vi "HDF5_append-dataset-Test4vi.vi"() -> ()   [LabVIEW 2018]
uses:
  <vilib>/addons/h5labview2/file/H5F.lvlib
  <vilib>/addons/h5labview2/file/H5Fmode.ctl
  <vilib>/addons/h5labview2/dataset/H5D.lvlib
  HDF5/HDF5_ToneInfoClust.ctl
  <vilib>/addons/h5labview2/dataset/H5Dwrite.llb/H5Dwrite.xnode
  <vilib>/addons/h5labview2/space/H5S.lvlib
  <vilib>/addons/h5labview2/base/H5Equery.vi
  HDF5/lib_path_mod_20200519.vi
  <vilib>/addons/h5labview2/dataset/H5Dread.llb/H5Dread.xnode
  <vilib>/addons/h5labview2/base/hid_t_renamed.ctl
panel:
  out "data 2":T1[](array[typedef])
  in  "data":i32[][](array[numeric])=[[0, 1, 2, 3, 4], [5, 6, 7, 8, 9]]
  out "ms/append":dbl
  out "timer (ms)":u32
  out "progress":i32(slide)=9999 scale=0.0..10.0
  in  "repetitions":i32=10
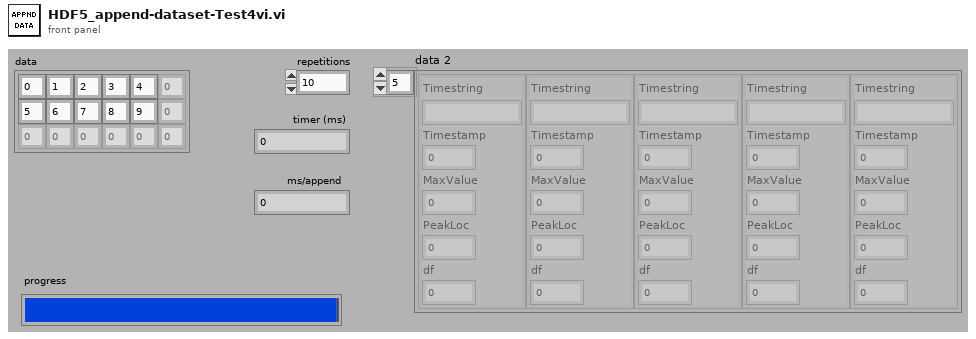
[diagram p1: front panel]
types:
  T1 = typedef "HDF5_ToneInfoClust.ctl" = cluster{"Timestring":string, "Timestamp":dbl, "MaxValue":dbl, "PeakLoc":dbl, "df":dbl}
  T2 = typedef "H5F.lvlib/H5Fmode.ctl" = enum16{"read-only", "read-write", "overwrite", "create new", "open or create"}
  T3 = typedef "HDF5_ToneInfoClust.ctl" = cluster{"Timestring":string, "Timestamp":timestamp, "MaxValue":dbl, "PeakLoc":dbl, "df":dbl}
  T4 = typedef "hid_t.ctl" = i32
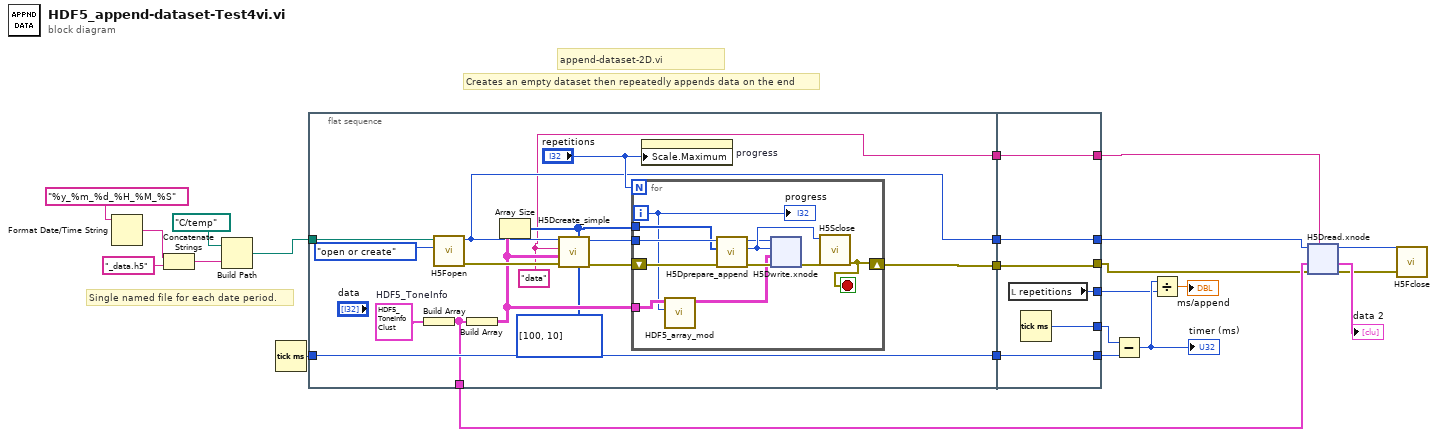
[diagram p0: block diagram]
diagram:
  # "Single named file for each date period."
  # "Creates an empty dataset then repeatedly appends data on the end"
  # "append-dataset-2D.vi"
  n1 = Format Date/Time String(time format string (%c)="%y_%m_%d_%H_%M_%S") -> (date/time string=w13:string)  [unwired: 2 in]
  n2 = Concatenate Strings(w13, "_data.h5" ("string")) -> (w15:string)
  n3 = Build Path(base path=path "C:/temp", name or relative path=w15) -> (appended path=w11:path)
  n4 = Tick Count (ms)() -> (millisecond timer value=w23:u32)
  n5 = flat-sequence {
    tunnel: w23 -> [w34]
    tunnel: [w34] -> w22
    tunnel: w11 -> [w32]
    tunnel: [w28] -> w9
    tunnel: [w27] -> w7
    tunnel: [w26] -> w6
    tunnel: [w25] -> w3
    tunnel: w22 -> [w73]
    tunnel: [w74] -> w21
    tunnel: [w73] -> w20
    tunnel: [w72] -> w18
    tunnel: [w71] -> w10
    tunnel: w9 -> [w71]
    tunnel: [w70] -> w8
    tunnel: w7 -> [w70]
    tunnel: [w69] -> w2
    tunnel: w3 -> [w69]
    frame #0 {
      w31 = T3 {"Timestring"="Timestamp string goes here", "Timestamp"=timestamp(0 s since 1904-01-01), "MaxValue"=0.0, "PeakLoc"=0.0, "df"=0.0}  # HDF5_ToneInfo
      w27 = "data" ("name")
      n6 = Build Array(w31) -> (w26:T3[])
      n7 = call <vilib>:"H5Fopen.vi"("mode (read-only)"=H5Fmode."open or create" ("mode"), "path"=w32) -> ("error out"=w35:errorcluster, "ref out"=w28:T4)  [unwired: 8 in]
      n8 = Build Array(w26) -> (w30:T3[][])
      n9 = Array Size(array=w30) -> (size(s)=w29:i32[])
      n10 = call <vilib>:"H5Dcreate_simple.vi"("max size"=u64[] [100, 10], "chunk size"=w29, "error in (no error)"=w35, "type in"=w30, "name"=w27, "ref in"=w28) -> ("error out"=w36:errorcluster, "dset out"=w37:T4)  [unwired: 4 in]
      n11 = for {
        N: "repetitions" -> [_]
        shift-right: [w45] -> w25
        shift-left: w36 -> [w46]
        tunnel: w29 -> [w47]
        tunnel: w37 -> [w48]
        tunnel: w30 -> [w41]
        i -> [w39]
        stop <- w45 stop-if-true
        n12 = call "HDF5_array_mod.vi"("delta"=w39, "Array in"=w41) -> ("Array out"=w40:T1[][])  [unwired: 9 in]
        n13 = call <vilib>:"H5Dprepare_append.vi"("error in (no error)"=w46, "append dims"=w47, "dset in"=w48) -> ("error out"=w49:errorcluster, "space out"=w43:T4, "dset out"=w42:T4)  [unwired: 5 in, 1 out]
        n14 = xnode "H5Dwrite.xnode"("error in (no error)"=w49, "data"=w40, "file space"=w43, "ref in"=w42) -> ("error out"=w44:errorcluster)  [unwired: 3 in, 2 out]
        n15 = call <vilib>:"H5Sclose.vi"("error in (no error)"=w44, "space in"=w43) -> ("error out"=w45:errorcluster)  [unwired: 9 in]
        "progress" <- w39
      }
      n16 = property on="progress" class="Slide (strict)"("Scale.Maximum"="repetitions") -> ()  [unwired: 2 in, 2 out]
    }
    frame #1 {
      n17 = local read "repetitions"() -> (w72:i32)
      n18 = Tick Count (ms)() -> (millisecond timer value=w74:u32)
    }
  }
  n19 = Subtract(x=w21, y=w20) -> (x-y=w19:u32)
  "timer (ms)" <- w19
  n20 = Divide(x=w19, y=w18) -> (x/y=→"ms/append":dbl)
  n21 = xnode "H5Dread.xnode"("dataset name (this)"=w8, "error in (no error)"=w2, "default"=w6, "ref in"=w10) -> ("error out"=w1:errorcluster, "data"=→"data 2":T3[], "ref out"=w5:i32)  [unwired: 2 in, 1 out]
  n22 = call <vilib>:"H5Fclose.vi"("error in (no error)"=w1, "ref"=w5) -> ()  [unwired: 9 in, 1 out]
